vi "VI_Heat_Tape_SubVI_Final_Final.vi"(8 "error in (no error)":errorcluster, 10 "Numeric":dbl, 11 "Modbus Master in":refnum<class "Modbus Master.lvclass">) -> (0 "error out":errorcluster, 3 "Modbus Master out":refnum<class "Modbus Master.lvclass">)   [LabVIEW 2019]
uses:
  <vilib>/NI/Modbus Library/API/Master/Modbus Master.lvclass
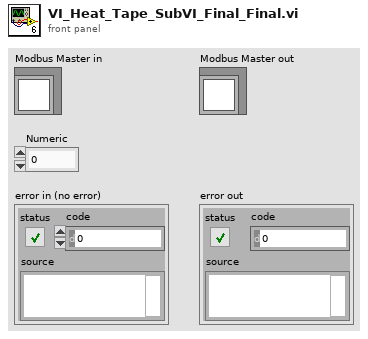
[diagram p1: front panel]
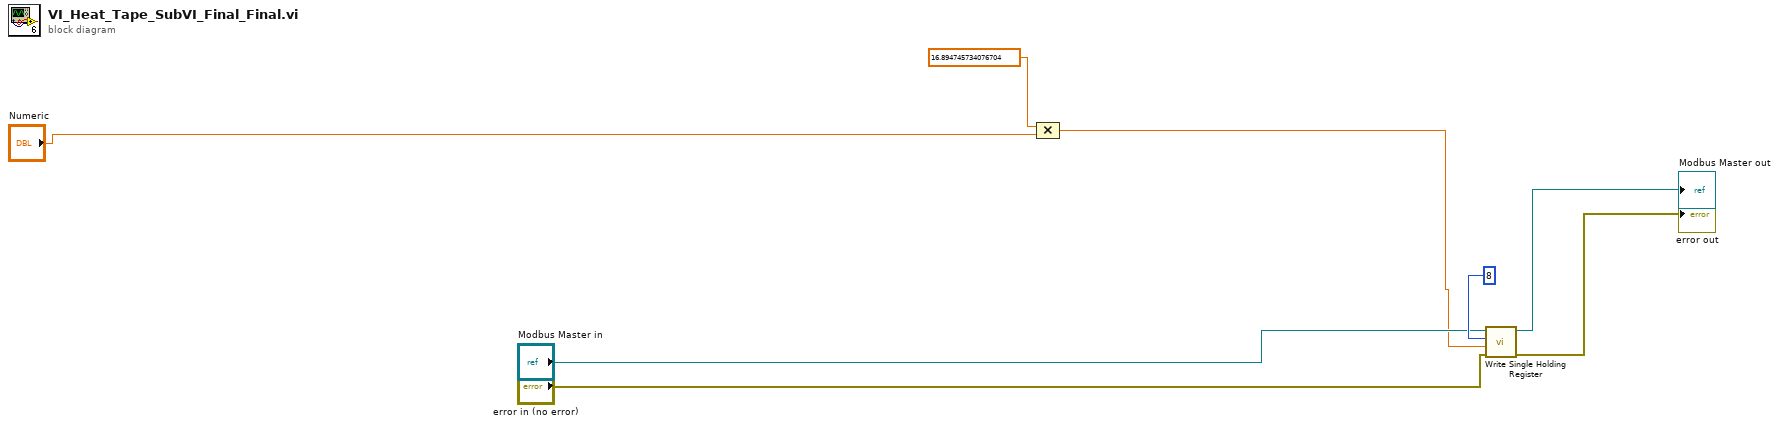
[diagram p0: block diagram]
diagram:
  n1 = Compound Arithmetic op=MULTIPLY(16.894745734076704 ("value"), "Numeric") -> (w2:dbl)
  n2 = call-dynamic "Write Single Holding Register.vi"("error in"="error in (no error)", "register to write"=w2, "address"=u16 8, "Modbus master in"="Modbus Master in") -> ("error out"=→"error out":errorcluster, "Modbus master out"=→"Modbus Master out":refnum<class "Modbus Master.lvclass">)  [unwired: 6 in]
